vi "SLSC Property Property Node.vi"   [LabVIEW 2020]
doc: "A Property Node with the SLSC Property class preselected. You must open the property using one of the Open Property VIs before you can use SLSC Property Property Node to query information about the property."
uses:
  <resource>/objmgr/slsc.rc
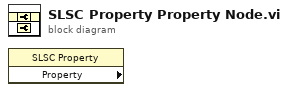
[diagram p0: block diagram]
diagram:
  n1 = property class="SLSC Property" props=[]() -> ()  [unwired: 2 in, 3 out]
